vi "failUnlessXmlParsedCorrectly.vi"(4 "Convert EOL? (TRUE)":bool=TRUE, 6 "message (\"\")":string, 8 "error in":errorcluster, 9 "Expected Data":variant, 10 "XML String":string, 11 "reference in":refnum<class "EasyXMLTest.lvclass">) -> (0 "error out":errorcluster, 2 "Produced Data":variant, 3 "reference in":refnum<class "EasyXMLTest.lvclass">)   [LabVIEW 2011, in "EasyXMLTest.lvclass"]
doc: "Tests whether an XML string input matches flattened XML output generated from an in data structure"
uses:
  EasyXMLTest.lvclass
panel:
  # "Copyright © 2007 James Kring, Inc. All rights reserved.\n\nAuthor: Jim Kring [jim.kring@jameskring.com]\n\nThis library is provided \"AS IS\" ,WITHOUT WARRANTIES OR \nCONDITIONS OF ANY KIND, either express or implied.\n\nJames Kring, Inc. -- http://www.jameskring.com"
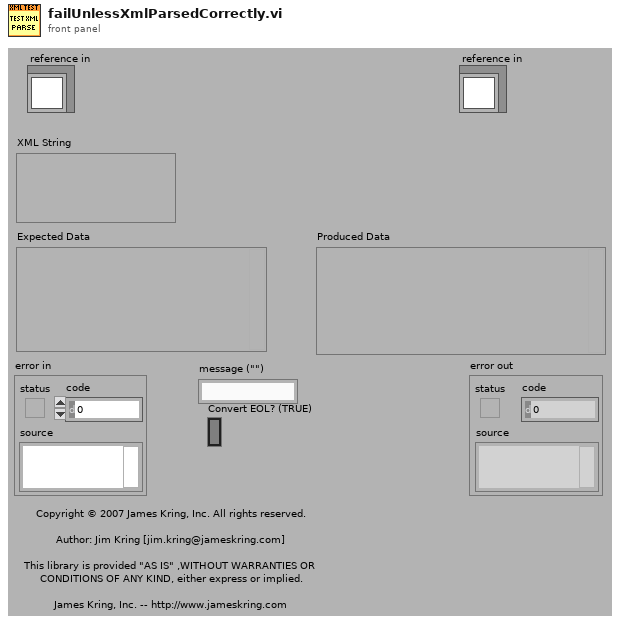
[diagram p1: front panel]
types:
  T1 = typedef "Type Descriptor__ogtk.ctl" = i16[]
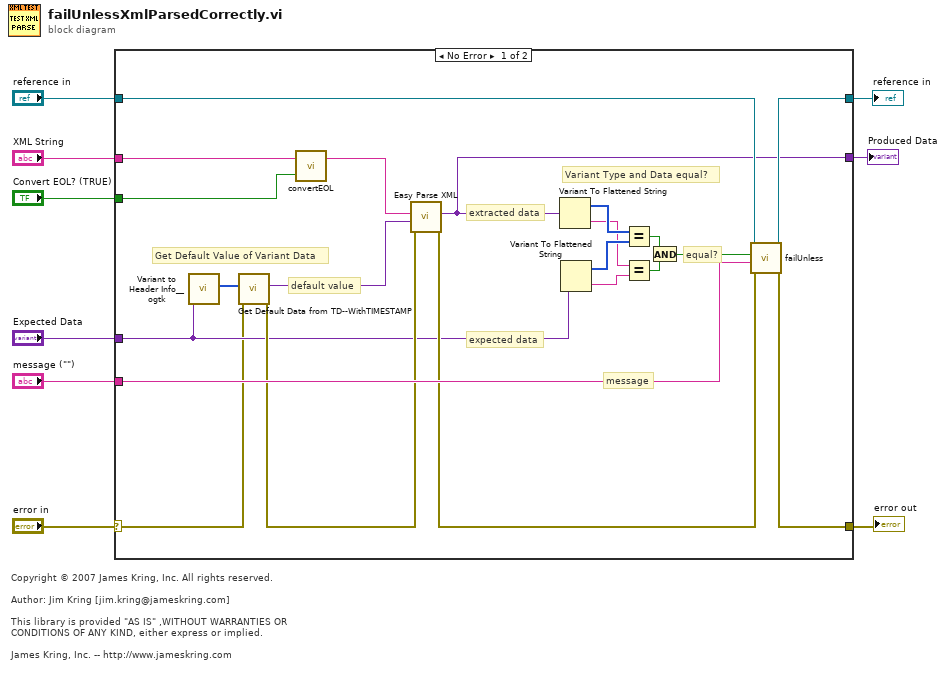
[diagram p0: block diagram]
diagram:
  # "Copyright © 2007 James Kring, Inc. All rights reserved.\n\nAuthor: Jim Kring [jim.kring@jameskring.com]\n\nThis library is provided \"AS IS\" ,WITHOUT WARRANTIES OR \nCONDITIONS OF ANY KIND, either express or implied.\n\nJames Kring, Inc. -- http://www.jameskring.com"
  n1 = case shown="No Error" "error in" {
    selector: "error in" -> [w10 w32]
    tunnel: [w24 w32] -> w8
    tunnel: [w26 w31] -> w6
    tunnel: "reference in" -> [w27 w31]
    tunnel: "message (\"\")" -> [w30 _]
    tunnel: "Expected Data" -> [w12 _]
    tunnel: "XML String" -> [w23 _]
    tunnel: [w20 _] -> w2
    tunnel: "Convert EOL? (TRUE)" -> [w21 _]
    frame No Error {
      # "Variant Type and Data equal?"
      # "message"
      # "equal?"
      # "expected data"
      # "extracted data"
      # "Get Default Value of Variant Data"
      # "default value"
      n2 = call <userlib>:"Variant to Header Info__ogtk.vi"("Variant"=w12) -> ("Type Descriptor"=w11:T1)  [unwired: 3 in, 2 out]
      n3 = call "Get Default Data from TD--WithTIMESTAMP.vi"("error in"=w10, "Type Descriptor"=w11) -> ("error out"=w29:errorcluster, "Default VData"=w28:variant)  [unwired: 8 in]
      n4 = call "convertEOL.vi"("Convert EOL? (TRUE)"=w21, "string"=w23) -> ("string out"=w22:string)  [unwired: 1 in]
      n5 = call "Easy Parse XML.vi"("error in (no error)"=w29, "LabVIEW Data (Type)"=w28, "XML String"=w22) -> ("error out"=w25:errorcluster, "LabVIEW Data"=w20:variant)  [unwired: 7 in]
      n6 = Variant To Flattened String(Variant=w20) -> (data string=w17:string, 1:w18:i16[])
      n7 = Variant To Flattened String(Variant=w12) -> (data string=w16:string, 1:w19:i16[])
      n8 = Equal?(x=w18, y=w19) -> (x = y?=w14:bool)
      n9 = Equal?(x=w17, y=w16) -> (x = y?=w15:bool)
      n10 = And(x=w14, y=w15) -> (x .and. y?=w13:bool)
      n11 = call-dynamic "failUnless.vi"("error in (no error)"=w25, "message (\"\")"=w30, "pass"=w13, "TestCase in"=w27) -> ("error out"=w24:errorcluster, "TestCase out"=w26:refnum<class "EasyXMLTest.lvclass">)  [unwired: 6 in]
    }
    frame Error {
    }
  }
  "error out" <- w8
  "reference in" <- w6
  "Produced Data" <- w2
